vi "patchparameters.vi"(1 "Params in":T1={"VC"=FALSE, "CC"=FALSE, "CC_icg (pA/mv)"=10.0, "VC_icg (mV/mV)"=10.0, "OCG (mV/pA)"=10.0, "OVG (mV/mV)"=10.0, "Vhold (mV)"=0.0, "holdon"=FALSE} {"Vhold (mV)" step=0.1 format="%_6g"; "OVG (mV/mV)" items=["2K"=2000.0, "1K"=1000.0, "500"=500.0, "200"=200.0, "100"=100.0, "50"=50.0, "20"=20.0, "10"=10.0, "5"=5.0, "2"=2.0, "1"=1.0, "0.5"=0.5, "0.2"=0.20000000298023224, "0.1"=0.10000000149011612, "0.05"=0.05000000074505806, "0.02"=0.019999999552965164, "0.01"=0.009999999776482582, "0.005"=0.004999999888241291]; "OCG (mV/pA)" items=["2K"=2000, "1K"=1000, "500"=500, "200"=200, "100"=100, "50"=50, "20"=20, "10"=10, "5"=5, "2"=2, "1"=1, "0.5"=0.5, "0.2"=0.2, "0.1"=0.1, "0.05"=0.05, "0.02"=0.02, "0.01"=0.01, "0.005"=0.005]; "VC_icg (mV/mV)" items=["0.1"=10]; "CC_icg (pA/mv)" items=["0.1"=10, "10"=0.1]}, 2 "command":string) -> (0 "Params out":T1={"VC"=FALSE, "CC"=FALSE, "CC_icg (pA/mv)"=10.0, "VC_icg (mV/mV)"=10.0, "OCG (mV/pA)"=10.0, "OVG (mV/mV)"=10.0, "Vhold (mV)"=0.0, "holdon"=FALSE} {"Vhold (mV)" step=0.1 format="%_6g"; "OVG (mV/mV)" items=["2K"=2000.0, "1K"=1000.0, "500"=500.0, "200"=200.0, "100"=100.0, "50"=50.0, "20"=20.0, "10"=10.0, "5"=5.0, "2"=2.0, "1"=1.0, "0.5"=0.5, "0.2"=0.20000000298023224, "0.1"=0.10000000149011612, "0.05"=0.05000000074505806, "0.02"=0.019999999552965164, "0.01"=0.009999999776482582, "0.005"=0.004999999888241291]; "OCG (mV/pA)" items=["2K"=2000, "1K"=1000, "500"=500, "200"=200, "100"=100, "50"=50, "20"=20, "10"=10, "5"=5, "2"=2, "1"=1, "0.5"=0.5, "0.2"=0.2, "0.1"=0.1, "0.05"=0.05, "0.02"=0.02, "0.01"=0.01, "0.005"=0.005]; "VC_icg (mV/mV)" items=["0.1"=10]; "CC_icg (pA/mv)" items=["0.1"=10, "10"=0.1]})   [LabVIEW 2015]
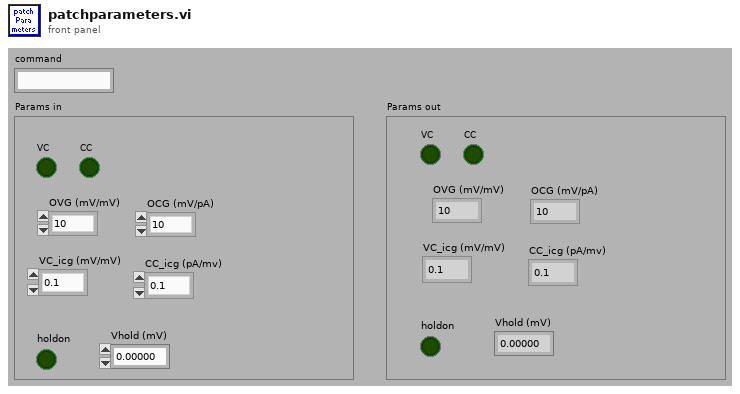
[diagram p1: front panel]
types:
  T1 = cluster{"VC":bool, "CC":bool, "CC_icg (pA/mv)":sgl, "VC_icg (mV/mV)":sgl, "OCG (mV/pA)":sgl, "OVG (mV/mV)":dbl, "Vhold (mV)":sgl, "holdon":bool}
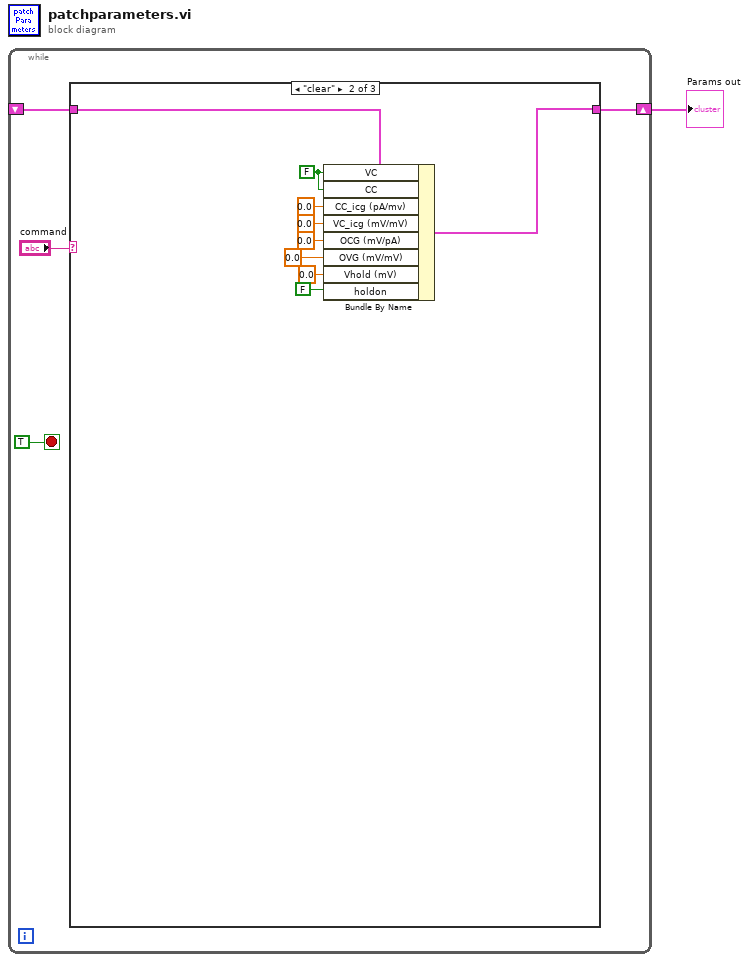
[diagram p0: block diagram]
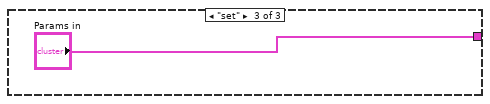
[diagram p3: hidden frame]
diagram:
  n1 = while {
    shift-right: [w3] -> w1
    shift-left: _ -> [w2]
    stop <- TRUE stop-if-true
    n2 = case shown="\"clear\"" "command" {
      tunnel: [w6 w7 "Params in"] -> w3
      tunnel: w2 -> [w6 w15 _]
      frame "get", Default {
      }
      frame "clear" {
        w14 = FALSE ("VC")
        n3 = Bundle By Name(cluster=w15, "VC"=w14, "CC"=w14, "CC_icg (pA/mv)"=0.0, "VC_icg (mV/mV)"=0.0, "OCG (mV/pA)"=0.0, "OVG (mV/mV)"=0.0, "Vhold (mV)"=0.0, "holdon"=FALSE) -> (w7:T1)
      }
      frame "set" {
      }
    }
  }
  "Params out" <- w1
